vi "Get Flip Vertical.vi"(8 "error in (no error)":errorcluster, 11 "senseHatDisplay in":refnum<class "RPI.SenseHat.Display.lvclass">) -> (0 "error out":errorcluster, 2 "Flip Vertical":bool, 3 "senseHatDisplay out":refnum<class "RPI.SenseHat.Display.lvclass">)   [LabVIEW 2020, in "RPI.SenseHat.Display.lvlib" / "RPI.SenseHat.Display.lvclass"]
doc: "Returns if we need to mirror the display vertically."
uses:
  RPI.SenseHat.Display.lvclass
  RPI.SenseHat.Display.lvclass/RPI.SenseHat.Display.ctl
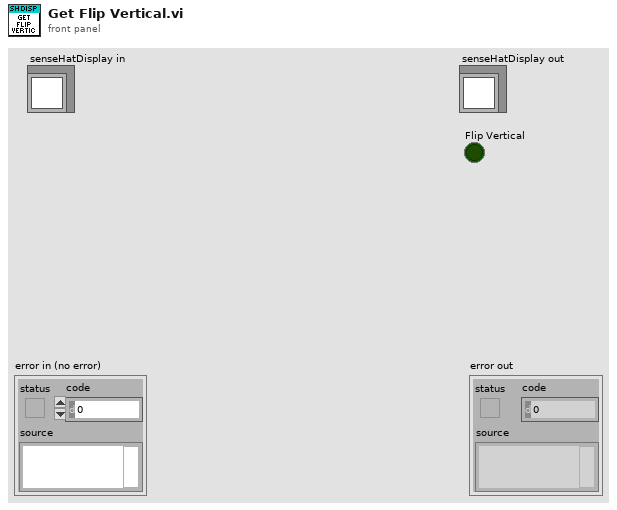
[diagram p1: front panel]
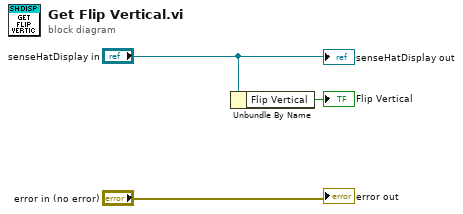
[diagram p0: block diagram]
diagram:
  n1 = Unbundle By Name("senseHatDisplay in") -> ("Flip Vertical"=→"Flip Vertical":bool)
  "error out" <- "error in (no error)"
  "senseHatDisplay out" <- "senseHatDisplay in"
